vi "Sample Transfer Initiate Stash.vi"(8 "error in (no error)":errorcluster, 11 "cRIO-CO2 in":refnum<class "cRIO-CO2.lvclass">) -> (0 "error out":errorcluster, 3 "cRIO-CO2 out":refnum<class "cRIO-CO2.lvclass">)   [LabVIEW 2015, in "cRIO-Carbondioxide.lvlib" / "cRIO-CO2.lvlib" / "cRIO-CO2.lvclass"]
uses:
  cRIO-CO2.lvclass
  cRIO-CO2.lvclass/cRIO-CO2.ctl
  Controls/Sample Transfer State Enumerator.ctl
  State Elapsed Time.vi
  Send Time-delayed Transfer Sample.vi
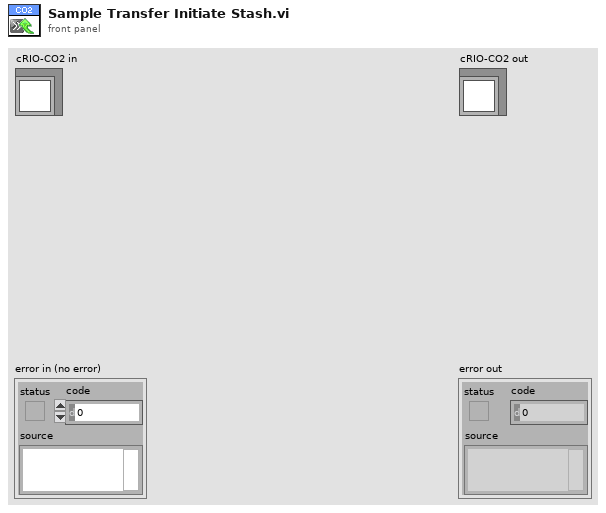
[diagram p1: front panel]
types:
  T1 = typedef "Sample Transfer State Enumerator.ctl" = enum16{"Idle", "Initialize", "Check Containers", "Check Temperatures", "Start Turbo", "Warm Up Containers", "Prepare for purging", "Purge Capillary", "Purge", "Open Containers", "Introduce Sample", "Measure Base Pressure", "Home Syringe", "Start Freezer", "Freeze Target", "Crystalize", "Initiate Stash", "Stash", "Polish", "Stop Freezers", "Push Sample", "Complete", "Abort", "Error", "Undefined"}
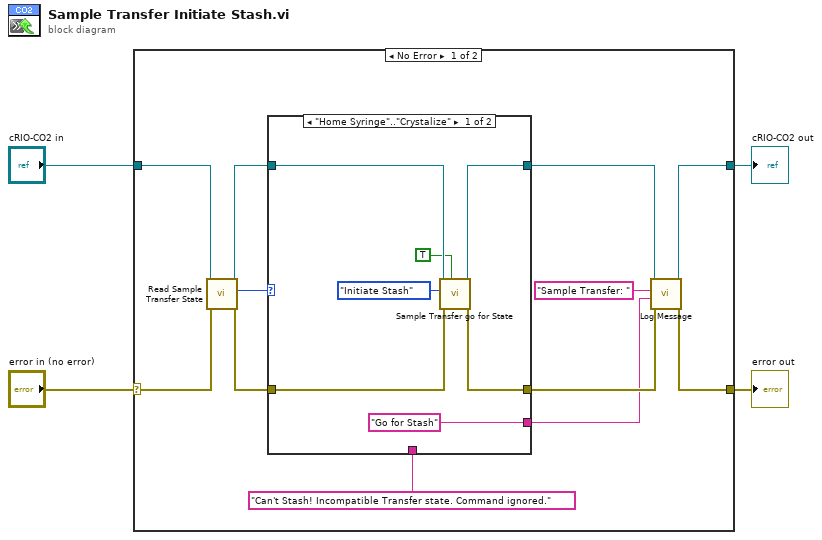
[diagram p0: block diagram]
diagram:
  n1 = case shown="No Error" "error in (no error)" {
    selector: "error in (no error)" -> [w16 w28]
    tunnel: [w10 w28] -> w3
    tunnel: [w8 w27] -> w1
    tunnel: "cRIO-CO2 in" -> [w15 w27]
    frame No Error {
      n2 = call "Read Sample Transfer State.vi"("error in (no error)"=w16, "cRIO-CO2 in"=w15) -> ("error out"=w5:errorcluster, "Sample Transfer State"=w13:T1, "cRIO-CO2 out"=w14:refnum<class "cRIO-CO2.lvclass">)  [unwired: 4 in, 3 out]
      n3 = case shown="\"Home Syringe\"..\"Crystalize\"" w13 {
        tunnel: w5 -> [w21 w25]
        tunnel: [w18 w25] -> w11
        tunnel: w14 -> [w20 w26]
        tunnel: [w17 w26] -> w9
        tunnel: ["Go for Stash" ("String") w24] -> w7
        tunnel: "Can't Stash! Incompatible Transfer state. Command ignored." ("String") -> [_ w24]
        frame "Home Syringe".."Crystalize" {
          n4 = call "Sample Transfer go for State.vi"("Restart Message (F)"=TRUE, "error in (no error)"=w21, "Sample Transfer State"=Sample_Transfer_State_Enumerator."Initiate Stash", "cRIO-CO2 in"=w20) -> ("error out"=w18:errorcluster, "cRIO-CO2 out"=w17:refnum<class "cRIO-CO2.lvclass">)  [unwired: 6 in]
        }
        frame Default {
        }
      }
      n5 = call "Log Message.vi"("error in (no error)"=w11, "String"=w7, "Source Name"="Sample Transfer: ", "cRIO-CO2 in"=w9) -> ("error out"=w10:errorcluster, "cRIO-CO2 out"=w8:refnum<class "cRIO-CO2.lvclass">)  [unwired: 6 in]
    }
    frame Error {
    }
  }
  "error out" <- w3
  "cRIO-CO2 out" <- w1
